vi "Dkm To Dxx.vi"(8 "error in (no error)":errorcluster, 10 "units":i32, 11 "dKilo":dbl) -> (0 "error out":errorcluster, 3 "dXX_Converted":dbl)   [LabVIEW 2024, in "POSCONV.lvlib"]
doc: "Converts double kilometres to any of the following units by setting the Units Control:\n\n1. case IN_MI:\n2. case IN_KM:\n3. case IN_M:\n4. case IN_ST:\n5. case IN_DMI:\n\n\n\n\n\ndouble DkmToDxx(double dKilo, int units);"
uses:
  POSCONV.lvlib
  POSCONV.dll
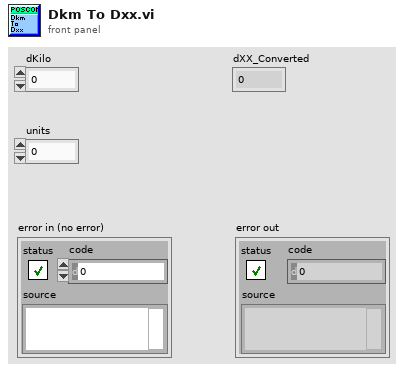
[diagram p1: front panel]
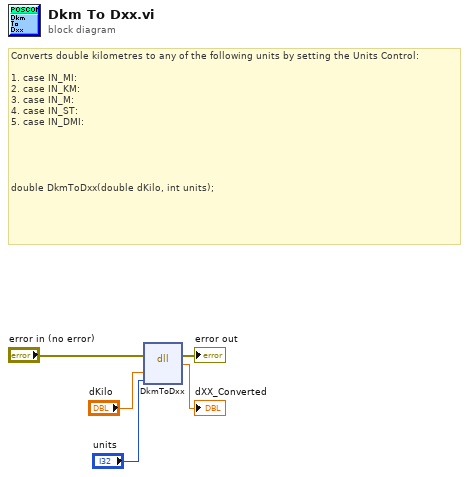
[diagram p0: block diagram]
diagram:
  # "Converts double kilometres to any of the following units by setting the Units Control:\n\n1. case IN_MI:\n2.\tcase IN_KM:\n3.\tcase IN_M:\n4.\tcase IN_ST:\n5.\tcase IN_DMI:\n\n\n\n\n\ndouble DkmToDxx(double dKilo, int units);"
  n1 = dll-call lib="C:/Users/Key-ES/Desktop/RailMeasurement_TVHR_SourceCode_v1.0.0_nonbatch/02 - Code/Modules/POSCONV/POSCONV.dll" fn="DkmToDxx"(error in="error in (no error)", "dKilo"="dKilo", "units"="units") -> (error out=→"error out":errorcluster, "return type"=→"dXX_Converted":dbl)  [unwired: 4 in, 1 out]
